vi "Log.vi"(7 "Source":string, 8 "error in (no error)":errorcluster, 9 "Message":string, 10 "Level":T1, 11 "Logging In":refnum<class "Logging.lvclass">) -> (0 "error out":errorcluster, 3 "Logging Out":refnum<class "Logging.lvclass">)   [LabVIEW 2020, in "Logging.lvclass"]
doc: "Enter a message into the system log."
uses:
  Logging.lvclass
  Level.ctl
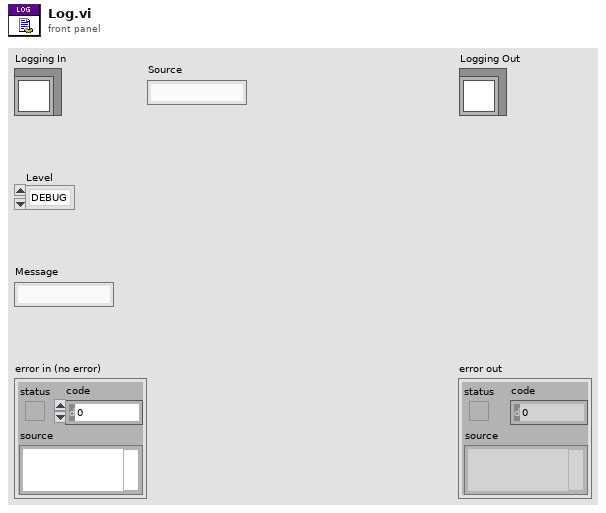
[diagram p1: front panel]
types:
  T1 = typedef "Logging.lvclass/Level.ctl" = enum16{"DEBUG", "INFO", "WARNING", "ERROR", "CRITICAL"}
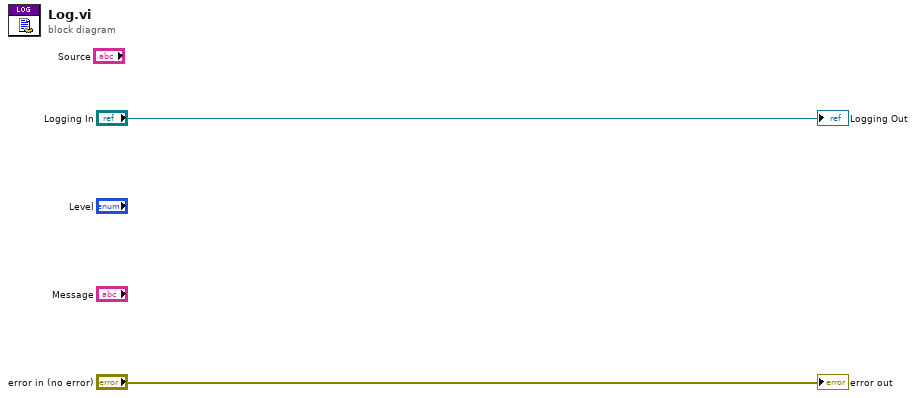
[diagram p0: block diagram]
diagram:
  "error out" <- "error in (no error)"
  "Logging Out" <- "Logging In"
